vi "Init.vi"(6 "ShadowColor":u32(colorbox)=9868950, 7 "Offset":i16, 8 "error in (no error)":errorcluster, 9 "Transparancy":i32, 10 "VI Refnum":refnum<vi>, 11 "Shadow in":refnum<class "Shadow.lvclass">) -> (0 "error out":errorcluster, 3 "Shadow out":refnum<class "Shadow.lvclass">)   [LabVIEW 2021, in "UIShadow.lvlib" / "Shadow.lvclass"]
uses:
  Shadow.lvclass
  Data.ctl
  Shadow.lvclass/Shadow.ctl
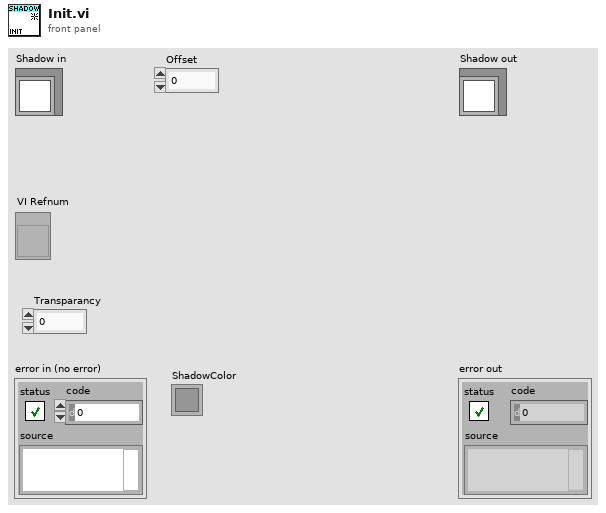
[diagram p1: front panel]
types:
  T1 = typedef "UIShadow.lvlib/Shadow.lvclass/Data.ctl" = cluster{"VI Refnum":refnum<vi>, "ShadowColor":u32, "Offset":i16, "Transparancy":i32, "UIShadowRef":refnum<vi>, "Activate?":bool}
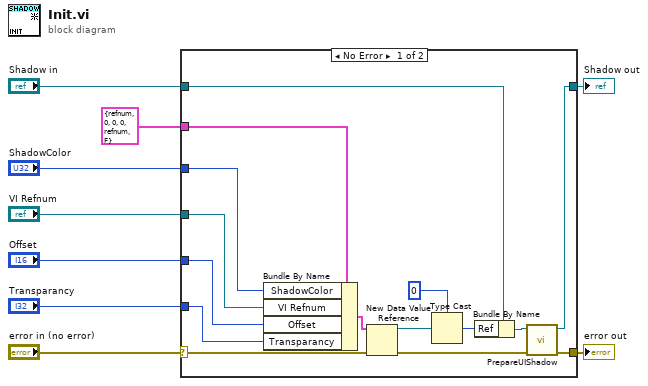
[diagram p0: block diagram]
diagram:
  n1 = case shown="No Error" "error in (no error)" {
    selector: "error in (no error)" -> [w24 w26]
    tunnel: [w19 w26] -> w8
    tunnel: [w21 w25] -> w6
    tunnel: "Shadow in" -> [w22 w25]
    tunnel: "VI Refnum" -> [w11 _]
    tunnel: T1 {"VI Refnum"=refnum, "ShadowColor"=0, "Offset"=0, "Transparancy"=0, "UIShadowRef"=refnum, "Activate?"=FALSE} ("Cluster") -> [w15 _]
    tunnel: "Transparancy" -> [w13 _]
    tunnel: "Offset" -> [w12 _]
    tunnel: "ShadowColor" -> [w10 _]
    frame No Error {
      n2 = Bundle By Name(cluster=w15, "ShadowColor"=w10, "VI Refnum"=w11, "Offset"=w12, "Transparancy"=w13) -> (w14:T1)
      n3 = New Data Value Reference(data value=w14, error in=w24) -> (data value reference=w23:refnum<data-value>, error out=w20:errorcluster)
      n4 = Type Cast(type=u64 0 ("Ref"), x=w23) -> (*(type *) &x=w16:u64)
      n5 = Bundle By Name(cluster=w22, "Ref"=w16) -> (w18:refnum<class "Shadow.lvclass">)
      n6 = call "PrepareUIShadow.vi"("error in (no error)"=w20, "Shadow in"=w18) -> ("error out"=w19:errorcluster, "Shadow out"=w21:refnum<class "Shadow.lvclass">)  [unwired: 8 in]
    }
    frame Error {
    }
  }
  "error out" <- w8
  "Shadow out" <- w6
